vi "Compute tau_phi & tau_m from Phasor.vi"(7 "max tau":dbl[unit], 8 "Error In":errorcluster, 9 "Call # (0)":i32, 10 "Phasor UCN[W] Parameters":T1, 11 "Phasor":cluster{"g":dbl, "s":dbl}) -> (0 "Error Out":errorcluster, 2 "tau_m":dbl[unit], 3 "tau_ph":dbl[unit])   [LabVIEW 2019]
uses:
  Phasor L_N[W] Parameters.ctl
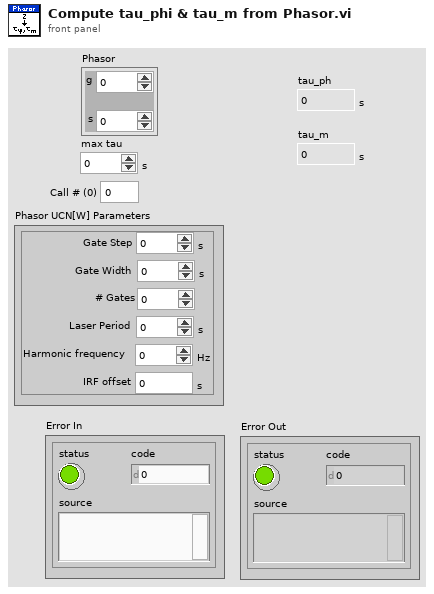
[diagram p1: front panel]
types:
  T1 = typedef "Phasor L_N[W] Parameters.ctl" = cluster{"Laser Period":dbl[unit], "Gate Width":dbl[unit], "Gate Step":dbl[unit], "Harmonic frequency":dbl[unit], "IRF offset":dbl[unit], "# Gates":dbl}
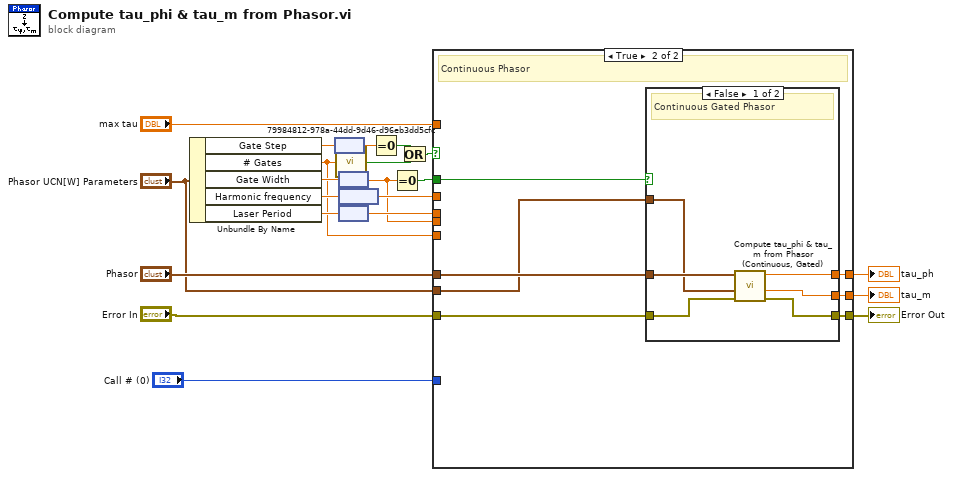
[diagram p0: block diagram]
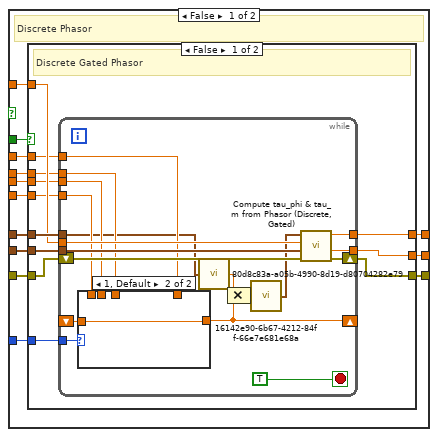
[diagram p2: hidden frame]
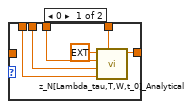
[diagram p3: hidden frame]
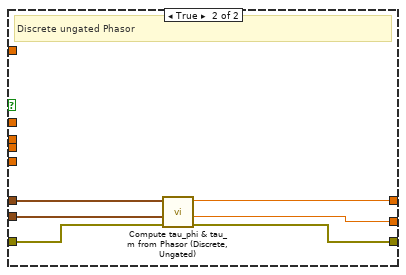
[diagram p4: hidden frame]
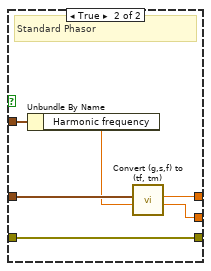
[diagram p5: hidden frame]
diagram:
  n1 = Unbundle By Name("Phasor UCN[W] Parameters") -> ("Gate Step"=w9:dbl[unit], "# Gates"=w1:dbl, "Gate Width"=w8:dbl[unit], "Harmonic frequency"=w6:dbl[unit], "Laser Period"=w4:dbl[unit])
  n2 = node(w9) -> (w21:dbl)
  n3 = call "79984812-978a-44dd-9d46-d96eb3dd5cfc.vi"("Number"=w1) -> ("Is NaN or Inf?"=w19:bool)  [unwired: 8 in]
  n4 = node(w8) -> (w2:dbl)
  n5 = node(w6) -> (w5:dbl)
  n6 = node(w4) -> (w3:dbl)
  n7 = Equal To 0?(x=w21) -> (x = 0?=w20:bool)
  n8 = Equal To 0?(x=w2) -> (x = 0?=w17:bool)
  n9 = Or(x=w20, y=w19) -> (x .or. y?=w18:bool)
  n10 = case shown="True" w18 {
    tunnel: w17 -> [w34 w84]
    tunnel: "Phasor" -> [w31 w83]
    tunnel: [w33 w82] -> w16
    tunnel: [w32 w81] -> w15
    tunnel: "max tau" -> [w30 _]
    tunnel: "Phasor UCN[W] Parameters" -> [w29 w78]
    tunnel: "Error In" -> [w28 w79]
    tunnel: [w27 w80] -> w11
    tunnel: "Call # (0)" -> [w26 _]
    tunnel: w5 -> [w25 _]
    tunnel: w3 -> [w24 _]
    tunnel: w2 -> [w23 _]
    tunnel: w1 -> [w22 _]
    frame False {
      # "Discrete Phasor"
      n11 = case shown="False" w34 {
        tunnel: [w46 w77] -> w33
        tunnel: [w45 w75] -> w32
        tunnel: w31 -> [w44 w76]
        tunnel: w30 -> [w43 _]
        tunnel: w29 -> [w42 w74]
        tunnel: w28 -> [w41 w73]
        tunnel: [w40 w72] -> w27
        tunnel: w26 -> [w39 _]
        tunnel: w25 -> [w38 _]
        tunnel: w24 -> [w37 _]
        tunnel: w23 -> [w36 _]
        tunnel: w22 -> [w35 _]
        frame False {
          # "Discrete Gated Phasor"
          n12 = while {
            tunnel: [w64] -> w46
            tunnel: [w63] -> w45
            tunnel: w44 -> [w52]
            tunnel: w43 -> [w62]
            tunnel: w42 -> [w61]
            shift-right: [w59] -> w40
            shift-left: w41 -> [w60]
            tunnel: w39 -> [w57]
            tunnel: w38 -> [w56]
            tunnel: w37 -> [w55]
            tunnel: w36 -> [w54]
            tunnel: w35 -> [w53]
            shift-right: [w50] -> _
            shift-left: _ -> [w49]
            stop <- TRUE stop-if-true
            n13 = case shown="1, Default" w57 {
              tunnel: w56 -> [w69 _]
              tunnel: w55 -> [w68 _]
              tunnel: w54 -> [w67 _]
              tunnel: w53 -> [w66 _]
              tunnel: [w65 w71] -> w50
              tunnel: w49 -> [_ w71]
              frame 0 {
                n14 = call "z_N[Lambda_tau,T,W,t_0]_Analytical.vi"("Harmonic f"=w69, "N"=w66, "W"=w67, "T"=w68, "tau"=ext 0.0) -> ("z_n,N,W(tau)"=w65:cxt)  [unwired: 6 in]
              }
              frame 1, Default {
              }
            }
            n15 = call "80d8c83a-a05b-4990-8d19-d80704282e79.vi"("Complex Coordinates"=w52) -> ("x + iy"=w51:cdb)  [unwired: 8 in]
            n16 = Compound Arithmetic op=MULTIPLY(w51, w50) -> (w48:cxt)
            n17 = call "16142e90-6b67-4212-84ff-66e7e681e68a.vi"("x + iy"=w48) -> ("Complex Coordinates"=w47:cluster{ext, ext})  [unwired: 8 in]
            n18 = call "Compute tau_phi & tau_m from Phasor (Discrete, Gated).vi"("Error In"=w60, "Phasor UCN[W] Parameters"=w61, "max tau"=w62, "Phasor"=w47) -> ("Error Out"=w59:errorcluster, "Modulus Lifetime"=w63:dbl[unit], "Phase Lifetime"=w64:dbl[unit])  [unwired: 3 in, 2 out]
          }
        }
        frame True {
          # "Discrete ungated Phasor"
          n19 = call "Compute tau_phi & tau_m from Phasor (Discrete, Ungated).vi"("Error In"=w73, "Phasor UCN[W] Parameters"=w74, "Phasor"=w76) -> ("Error Out"=w72:errorcluster, "Modulus Lifetime"=w75:dbl[unit], "Phase Lifetime"=w77:dbl[unit])  [unwired: 6 in]
        }
      }
    }
    frame True {
      # "Continuous Phasor"
      n20 = case shown="False" w84 {
        tunnel: w83 -> [w88 w96]
        tunnel: [w90 w95] -> w82
        tunnel: [w89 w94] -> w81
        tunnel: [w85 w93] -> w80
        tunnel: w79 -> [w86 w93]
        tunnel: w78 -> [w87 w92]
        frame False {
          # "Continuous Gated Phasor"
          n21 = call "Compute tau_phi & tau_m from Phasor (Continuous, Gated).vi"("Error In"=w86, "Phasor UCN[W] Parameters"=w87, "Phasor"=w88) -> ("Error Out"=w85:errorcluster, "Modulus Lifetime"=w89:dbl[unit], "Phase Lifetime"=w90:dbl[unit])  [unwired: 6 in]
        }
        frame True {
          # "Standard Phasor"
          n22 = Unbundle By Name(w92) -> ("Harmonic frequency"=w91:dbl[unit])
          n23 = call "Convert (g,s,f) to (tf, tm).vi"("Phasor Harmonic Frequency"=w91, "Phasor (g, s)"=w96) -> ("Modulus Lifetime"=w94:dbl[unit], "Phase Lifetime"=w95:dbl[unit])  [unwired: 8 in]
        }
      }
    }
  }
  "tau_m" <- w15
  "tau_ph" <- w16
  "Error Out" <- w11
